vi "Shut_down_heated_tunnel.vi"(3 "Mode":T5, 5 "Traverse line In":T2 {"Row Duration (mins)" format="%#.1f"; "Row No" min=0; "Trace Gas Concentration (%)" min=0.0 format="%#.2f"; "Emission Rate (l/min)" format="%#.2f"; "Tunnel Speed" format="%#.2f"; "Start X" format="%#.2f"; "Start Y" format="%#.2f"; "Start Z" format="%#.2f"; "End X" format="%#.2f"; "End Y" format="%#.2f"; "End Z" format="%#.2f"; "Averaging time (min)" min=0.0 format="%#.1f"}) -> (0 "Error Message":string, 1 "Status":T1, 2 "Traverse line Out":T2 {"Row Duration (mins)" format="%#.1f"; "Row No" min=0; "Trace Gas Concentration (%)" min=0.0 format="%#.2f"; "Emission Rate (l/min)" format="%#.2f"; "Tunnel Speed" format="%#.2f"; "Start X" format="%#.2f"; "Start Y" format="%#.2f"; "Start Z" format="%#.2f"; "End X" format="%#.2f"; "End Y" format="%#.2f"; "End Z" format="%#.2f"; "Averaging time (min)" min=0.0 format="%#.1f"})   [LabVIEW 2010]
uses:
  Gen Trav/Traverse_cluster.ctl
  Gen Trav/Spacing.ctl
  Controls/Multi_run_mode.ctl
  Controls/User_Specific_mode.ctl
  Gen Trav/Multi_Run_Status.ctl
  ADAM Client/Sub VIs/ADAM Controls/Update_scan_value.ctl
panel:
  # "X           Y            Z"
  # "Start"
  # "End"
  # "X           Y            Z"
  # "Start"
  # "End"
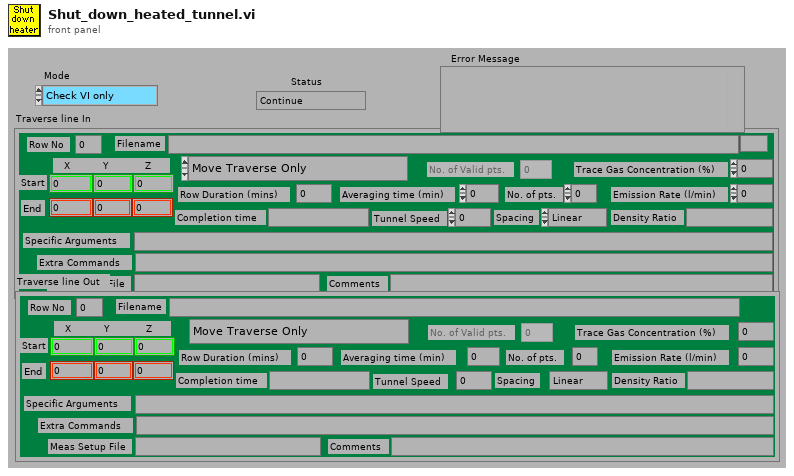
[diagram p1: front panel]
types:
  T1 = typedef "Multi_Run_Status.ctl" = enum16{"Continue", "Jump to Next Point", "Jump to Next Row", "Jump To Fall Back", "Terminate Run"}
  T2 = typedef "Traverse_cluster.ctl" = cluster{"Start X":dbl, "Start Y":dbl, "Start Z":dbl, "End X":dbl, "End Y":dbl, "End Z":dbl, "No. of pts.":i32, "Spacing":T3, "Filename":path, "Tunnel Speed":dbl, "Averaging time (min)":dbl, "Extra Commands":string, "Specific Arguments":string, "Emission Rate (l/min)":dbl, "Trace Gas Concentration (%)":dbl, "Density Ratio":string, "Comments":string, "Row No":i32, "Row Type Selector":T4, "Completion time":string, "Row Duration (mins)":dbl, "No. of Valid pts.":i32, "Meas Setup File":string}
  T3 = typedef "Spacing.ctl" = enum16{"Linear", "Log", "Gauss", "Specified", "N/A"}
  T4 = typedef "Multi_run_mode.ctl" = enum16{"Move Traverse Only", "Set Tunnel Speed Only", "Set Source Only", "Set Measurement Conditions", "Single Measurement", "Vertical Profile", "Lateral Profile", "Longitudinal Profile", "Explore Volume", "Multi-Axis Profile", "Auto Calibrate", "Meas Fast FID Bkgnd", "Check Beam Power", "Scanning Valve Measurement", "Run VI Named:", "Set ADAM Ch", "Wait (minutes)", "Send Message", "Synchronize With:", "Fall Back to this Row", "Turn Off Row Repeating", "Blank Row"}
  T5 = typedef "User_Specific_mode.ctl" = enum16{"Check VI only", "Run VI"}
  T6 = typedef "Update_scan_value.ctl" = cluster{"Channel Name":string, "New Value":dbl}
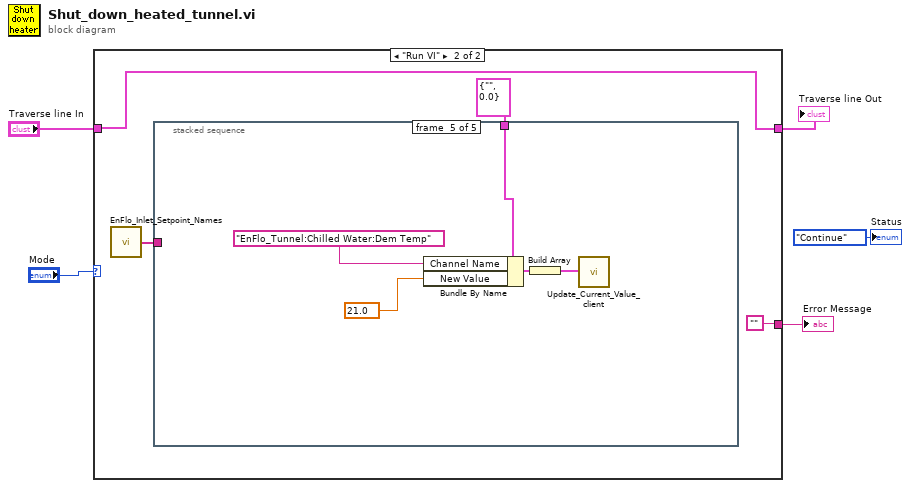
[diagram p0: block diagram]
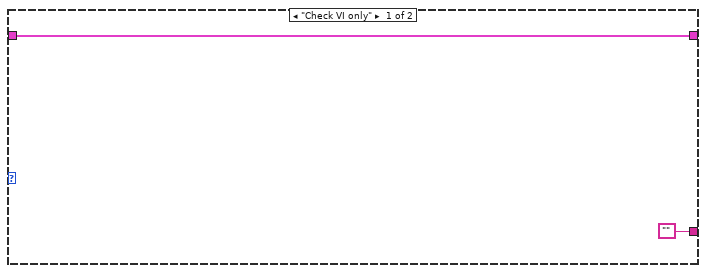
[diagram p2: hidden frame]
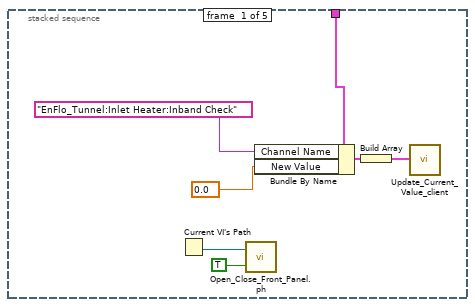
[diagram p3: hidden frame]
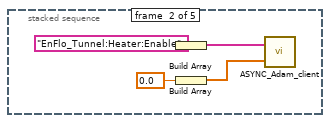
[diagram p4: hidden frame]
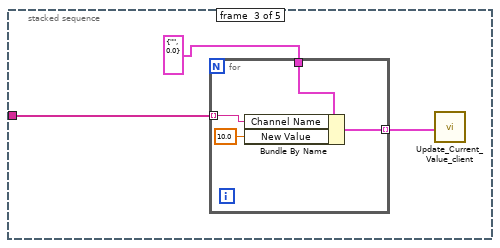
[diagram p5: hidden frame]
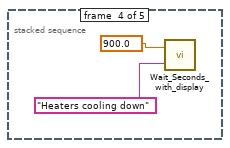
[diagram p6: hidden frame]
diagram:
  n1 = case shown="\"Run VI\"" "Mode" {
    tunnel: "Traverse line In" -> [w7 w10]
    tunnel: [w7 w10] -> w3
    tunnel: ["" ""] -> w2
    frame "Check VI only" {
    }
    frame "Run VI" {
      n2 = call "EnFlo_Inlet_Setpoint_Names.vi"() -> ("Sub Names"=w9:string[])
      n3 = stacked-sequence {
        tunnel: T6 {"Channel Name"="", "New Value"=0.0} ("Update Scan Value Cluster") -> [w14 _ _ _ w32]
        tunnel: w9 -> [_ _ w24 _ _]
        frame #0 {
          n4 = Current VI's Path() -> (path=w12:path)
          n5 = call "Open_Close_Front_Panel.ph.vi"("Front Panel Window:Open"=TRUE, "VI path"=w12) -> ()  [unwired: 2 out]
          n6 = Bundle By Name(cluster=w14, "Channel Name"="EnFlo_Tunnel:Inlet Heater:Inband Check", "New Value"=0.0 ("Bundle Element")) -> (w17:T6)
          n7 = Build Array(w17) -> (w16:T6[])
          n8 = call "Update_Current_Value_client.vi"("Update array in"=w16) -> ()  [unwired: 1 in]
        }
        frame #1 {
          n9 = Build Array("EnFlo_Tunnel:Heater:Enable") -> (w22:string[])
          n10 = Build Array(0.0 ("Input Element")) -> (w19:dbl[])
          n11 = call "ASYNC_Adam_client.vi"("Values"=w19, "Channel Names"=w22) -> ()  [unwired: 2 out]
        }
        frame #2 {
          n12 = for {
            tunnel: T6 {"Channel Name"="", "New Value"=0.0} ("Update Scan Value Cluster") -> [w29]
            tunnel: w24 -> [w28] mode=indexing
            tunnel: [w26] -> w23 mode=indexing
            n13 = Bundle By Name(cluster=w29, "Channel Name"=w28, "New Value"=10.0) -> (w26:T6)
          }
          n14 = call "Update_Current_Value_client.vi"("Update array in"=w23) -> ()  [unwired: 1 in]
        }
        frame #3 {
          n15 = call "Wait_Seconds_with_display.vi"("Message"="Heaters cooling down", "Seconds to wait"=900.0) -> ()  [unwired: 2 out]
        }
        frame #4 {
          n16 = Bundle By Name(cluster=w32, "Channel Name"="EnFlo_Tunnel:Chilled Water:Dem Temp", "New Value"=21.0 ("Bundle Element")) -> (w35:T6)
          n17 = Build Array(w35) -> (w34:T6[])
          n18 = call "Update_Current_Value_client.vi"("Update array in"=w34) -> ()  [unwired: 1 in]
        }
      }
    }
  }
  "Traverse line Out" <- w3
  "Error Message" <- w2
  "Status" <- Multi_Run_Status."Continue" ("Status")
